vi "CalVEIN Main FRANK SFT.vi"() -> ()   [LabVIEW 2016]
uses:
  Type Defs/Sensor Data.ctl
  Type Defs/Boxcar.ctl
  Control 1.ctl
panel:
  out "MV FUEL PT":T1="-1.97 psig"
  out "MV LOX PT":string="-1.37 psig"
  out "45% 2":string="27.30 °C"
  out "45%":string="27.40 °C"
  in  "Box cooler":bool
  out "NewVal":bool
  out "Ready To Fire Flag":bool
  out "Firing State":string[](array[string])=["System Is Not Armed", "  \n", " ", " ", " ", " ", " ", " "]
  in  "Arm Flag":bool
  in  "Sample Rate (secs)":u32=1000
  out "Burn Time\nCountdown (secs)":string="0.00"
  out "Boxcar Data":T2={"AI Sensor Data"={"Sensor Array"=[{"Description"="MV FUEL PT", "Last Reading"="-1.37", "Coefs"=[0.0, 5000.0], "Eng Units"="psig"}, {"Description"="MV FUEL PT", "Last Reading"="-1.97", "Coefs"=[0.0, 5000.0], "Eng Units"="psig"}, {"Description"="P1 - Chamber Pressure", "Last Reading"="-1.37", "Coefs"=[0.0, 5000.0], "Eng Units"="psig"}, {"Description"="Not Used", "Last Reading"="0.00", "Coefs"=[0.0, 0.0], "Eng Units"="psig"}, {"Description"="High Press", "Last Reading"="141.40", "Coefs"=[157.22, 50099.0], "Eng Units"="psig"}, {"Description"="Not Use", "Last Reading"="0.00", "Coefs"=[0.0, 0.0], "Eng Units"="psig"}, {"Description"="Load Cell", "Last Reading"="-5.59", "Coefs"=[-8.51, -8297.0], "Eng Units"="lb"}, {"Description"="CHAMBER", "Last Reading"="-0.98", "Coefs"=[0.0, 5000.0], "Eng Units"="psig"}, {"Description"="P6 - GHE Fill Pressure", "Last Reading"="-0.32", "Coefs"=[0.0, 5000.0], "Eng Units"="psig"}, {"Description"="P8 - Pneumatics Pressure", "Last Reading"="-0.78", "Coefs"=[0.0, 5000.0], "Eng Units"="psig"}, {"Description"="Not Used", "Last Reading"="0.00", "Coefs"=[0.0, 0.0], "Eng Units"=""}, {"Description"="Not Used", "Last Reading"="0.00", "Coefs"=[0.0, 0.0], "Eng Units"=""}, {"Description"="Not Used", "Last Reading"="0.00", "Coefs"=[0.0, 0.0], "Eng Units"=""}, {"Description"="Not Used", "Last Reading"="0.00", "Coefs"=[0.0, 0.0], "Eng Units"=""}, {"Description"="Not Used", "Last Reading"="0.00", "Coefs"=[0.0, 0.0], "Eng Units"=""}, {"Description"="Not Used", "Last Reading"="0.00", "Coefs"=[0.0, 0.0], "Eng Units"=""}, {"Description"="QD Sep Indication", "Last Reading"="5.11", "Coefs"=[0.0, 1.0], "Eng Units"="On/Off"}, {"Description"="Lift Off Indicator", "Last Reading"="5.11", "Coefs"=[0.0, 1.0], "Eng Units"="On/Off"}, {"Description"="Main Valve Open Indicator", "Last Reading"="1.73", "Coefs"=[0.0, 1.0], "Eng Units"="On/Off"}, {"Description"="Main Valve Closed Indicator", "Last Reading"="1.68", "Coefs"=[0.0, 1.0], "Eng Units"="On/Off"}, {"Description"="Load Cell 1 - Veh Gross Weight", "Last Reading"="-17.67", "Coefs"=[-122.0, 8333.3], "Eng Units"="lbf"}, {"Description"="Load Cell 2 - - Veh Gross Weight", "Last Reading"="-2.48", "Coefs"=[0.0, 8333.33], "Eng Units"="lbf"}, {"Description"="Not Used", "Last Reading"="0.00", "Coefs"=[0.0, 0.0], "Eng Units"=""}, {"Description"="Not Used", "Last Reading"="0.00", "Coefs"=[0.0, 0.0], "Eng Units"=""}, {"Description"="LOX TANK SFT ", "Last Reading"="-126.56", "Coefs"=[-126.49, 245.99], "Eng Units"="psi"}, {"Description"="FUEL TANK SFT ", "Last Reading"="-126.56", "Coefs"=[-126.49, 245.99], "Eng Units"="psi"}, {"Description"="DOME SET SFT", "Last Reading"="-126.56", "Coefs"=[-126.49, 245.99], "Eng Units"="psi"}, {"Description"="", "Last Reading"="0.00", "Coefs"=[], "Eng Units"=""}, {"Description"="", "Last Reading"="0.00", "Coefs"=[], "Eng Units"=""}, {"Description"="", "Last Reading"="0.00", "Coefs"=[], "Eng Units"=""}, {"Description"="", "Last Reading"="0.00", "Coefs"=[], "Eng Units"=""}, {"Description"="", "Last Reading"="0.00", "Coefs"=[], "Eng Units"=""}]}, "TC Array"=[27.395629361000005, 27.395629361000005, 27.395629361000005, 27.2964472325, 27.494811489499995, 27.395629361000005, 27.395629361000005, 1369.6815, 1369.6815, 1369.6815, 1369.6815, 1369.6815, 1369.6815, 1369.6815]}
  out "?":string="-0.32 psig"
  out "Log Refnum":refnum<file>
  out "Log Epoch":u32
  out "Log Number":i32=279
  in  "Data Log Flag":bool
  out "File Path":path
  out "Eng Data & Units":string[](array[string])=["-1.37 psig", "-1.97 psig", "-1.33 psig", "0.00 psig", "141.40 psig", "0.00 psig", "-5.59 lb", "-0.98 psig", "-0.32 psig", "-0.73 psig", "0.00 ", "0.00 ", "0.00 ", "0.00 ", "0.00 ", "0.00 ", "5.10 On/Off", "5.11 On/Off", "1.73 On/Off", "1.69 On/Off", "-17.67 lbf", "-2.48 lbf", "0.00 ", "0.00 ", "-126.56 psi", "-126.56 psi", "-126.56 psi", "0.00 ", "0.00 ", "0.00 ", "0.00 ", "0.00 "]
  out "TC String Array":string[](array[string])=["27.40 °C", "27.40 °C", "27.40 °C", "27.30 °C", "27.49 °C", "27.40 °C", "27.40 °C", "1369.68 °C", "1369.68 °C", "1369.68 °C", "1369.68 °C", "1369.68 °C", "1369.68 °C", "1369.68 °C"]
  in  "Data Log Button":bool
  in  "Sequence Abort":bool
  out "Igniter Abort":bool
  out "Elapsed Time":u32=10554
  in  "Auto Sequence":bool
  in  "Auto Sequence Flag":bool
  out "Epoch":u32=5746771
  out "Countdown (secs)":i32
  in  "MV Open Start":dbl
  in  "Burn Time":dbl=300.0
  in  "Igniter Start":dbl=-3.0
  in  "Countdown":dbl=-10.0
  in  "Igniter Minimum\nTemp (°C)":dbl=100.0
  in  "Auto Switch":bool
  out "?":string="1369.68 °C"
  out "Thermometer 2":dbl(slide)=1369.6815 scale=0.0..1000.0
  out "Thermometer":dbl(slide)=1369.6815 scale=0.0..1000.0
  out "Igniter Temp (°C)":string="1369.68 °C"
  out "?":string="27.40 °C"
  out "30%":string="27.40 °C"
  out "QD Sep Indicator":bool=TRUE
  out "Liftoff Indicator":bool=TRUE
  out "MV Closed Ind":bool
  out "MV Open Ind":bool
  out "Load Cell":string="-5.59 lb"
  out "?":string="-0.73 psig"
  out "?":string="-0.98 psig"
  out "?":string="-126.56 psi"
  out "?":string="141.40 psig"
  out "?":string="-0.98 psig"
  out "P3":string="-126.56 psi"
  in  "High Press":bool
  in  "High Press Vent":bool
  in  "MV Open":bool
  in  "MV Closed":bool
  out "P2":string="-126.56 psi"
  in  "Remote QD Sep":bool
  in  "GHe Fill":bool
  in  "Igniter Pwr":bool
  in  "Dome Set":bool
  in  "Dome Vent":bool
  in  "Fuel Vent":bool
  in  "LOX Vent":bool
  out "Relay States":bool[](array[boolean])
  in  "stop":bool
  in  "AI Sensor Data":T3={"Sensor Array"=[{"Description"="MV FUEL PT", "Last Reading"="-1.37", "Coefs"=[0.0, 5000.0], "Eng Units"="psig"}, {"Description"="MV FUEL PT", "Last Reading"="-1.97", "Coefs"=[0.0, 5000.0], "Eng Units"="psig"}, {"Description"="P1 - Chamber Pressure", "Last Reading"="-1.33", "Coefs"=[0.0, 5000.0], "Eng Units"="psig"}, {"Description"="Not Used", "Last Reading"="0.00", "Coefs"=[0.0, 0.0], "Eng Units"="psig"}, {"Description"="High Press", "Last Reading"="141.40", "Coefs"=[157.22, 50099.0], "Eng Units"="psig"}, {"Description"="Not Use", "Last Reading"="0.00", "Coefs"=[0.0, 0.0], "Eng Units"="psig"}, {"Description"="Load Cell", "Last Reading"="-5.59", "Coefs"=[-8.51, -8297.0], "Eng Units"="lb"}, {"Description"="CHAMBER", "Last Reading"="-0.98", "Coefs"=[0.0, 5000.0], "Eng Units"="psig"}, {"Description"="P6 - GHE Fill Pressure", "Last Reading"="-0.32", "Coefs"=[0.0, 5000.0], "Eng Units"="psig"}, {"Description"="P8 - Pneumatics Pressure", "Last Reading"="-0.73", "Coefs"=[0.0, 5000.0], "Eng Units"="psig"}, {"Description"="Not Used", "Last Reading"="0.00", "Coefs"=[0.0, 0.0], "Eng Units"=""}, {"Description"="Not Used", "Last Reading"="0.00", "Coefs"=[0.0, 0.0], "Eng Units"=""}, {"Description"="Not Used", "Last Reading"="0.00", "Coefs"=[0.0, 0.0], "Eng Units"=""}, {"Description"="Not Used", "Last Reading"="0.00", "Coefs"=[0.0, 0.0], "Eng Units"=""}, {"Description"="Not Used", "Last Reading"="0.00", "Coefs"=[0.0, 0.0], "Eng Units"=""}, {"Description"="Not Used", "Last Reading"="0.00", "Coefs"=[0.0, 0.0], "Eng Units"=""}, {"Description"="QD Sep Indication", "Last Reading"="5.10", "Coefs"=[0.0, 1.0], "Eng Units"="On/Off"}, {"Description"="Lift Off Indicator", "Last Reading"="5.11", "Coefs"=[0.0, 1.0], "Eng Units"="On/Off"}, {"Description"="Main Valve Open Indicator", "Last Reading"="1.73", "Coefs"=[0.0, 1.0], "Eng Units"="On/Off"}, {"Description"="Main Valve Closed Indicator", "Last Reading"="1.69", "Coefs"=[0.0, 1.0], "Eng Units"="On/Off"}, {"Description"="Load Cell 1 - Veh Gross Weight", "Last Reading"="-17.67", "Coefs"=[-122.0, 8333.3], "Eng Units"="lbf"}, {"Description"="Load Cell 2 - - Veh Gross Weight", "Last Reading"="-2.48", "Coefs"=[0.0, 8333.33], "Eng Units"="lbf"}, {"Description"="Not Used", "Last Reading"="0.00", "Coefs"=[0.0, 0.0], "Eng Units"=""}, {"Description"="Not Used", "Last Reading"="0.00", "Coefs"=[0.0, 0.0], "Eng Units"=""}, {"Description"="LOX TANK SFT ", "Last Reading"="-126.56", "Coefs"=[-126.49, 245.99], "Eng Units"="psi"}, {"Description"="FUEL TANK SFT ", "Last Reading"="-126.56", "Coefs"=[-126.49, 245.99], "Eng Units"="psi"}, {"Description"="DOME SET SFT", "Last Reading"="-126.56", "Coefs"=[-126.49, 245.99], "Eng Units"="psi"}, {"Description"="", "Last Reading"="0.00", "Coefs"=[], "Eng Units"=""}, {"Description"="", "Last Reading"="0.00", "Coefs"=[], "Eng Units"=""}, {"Description"="", "Last Reading"="0.00", "Coefs"=[], "Eng Units"=""}, {"Description"="", "Last Reading"="0.00", "Coefs"=[], "Eng Units"=""}, {"Description"="", "Last Reading"="0.00", "Coefs"=[], "Eng Units"=""}]}
  # "CSULB Launch Team Control System"
  # "Questions regrads this system please direct them to Thanh Truc Le truclee126@gmail.com"
  # "Autosequence\n Parameters"
  # "30%"
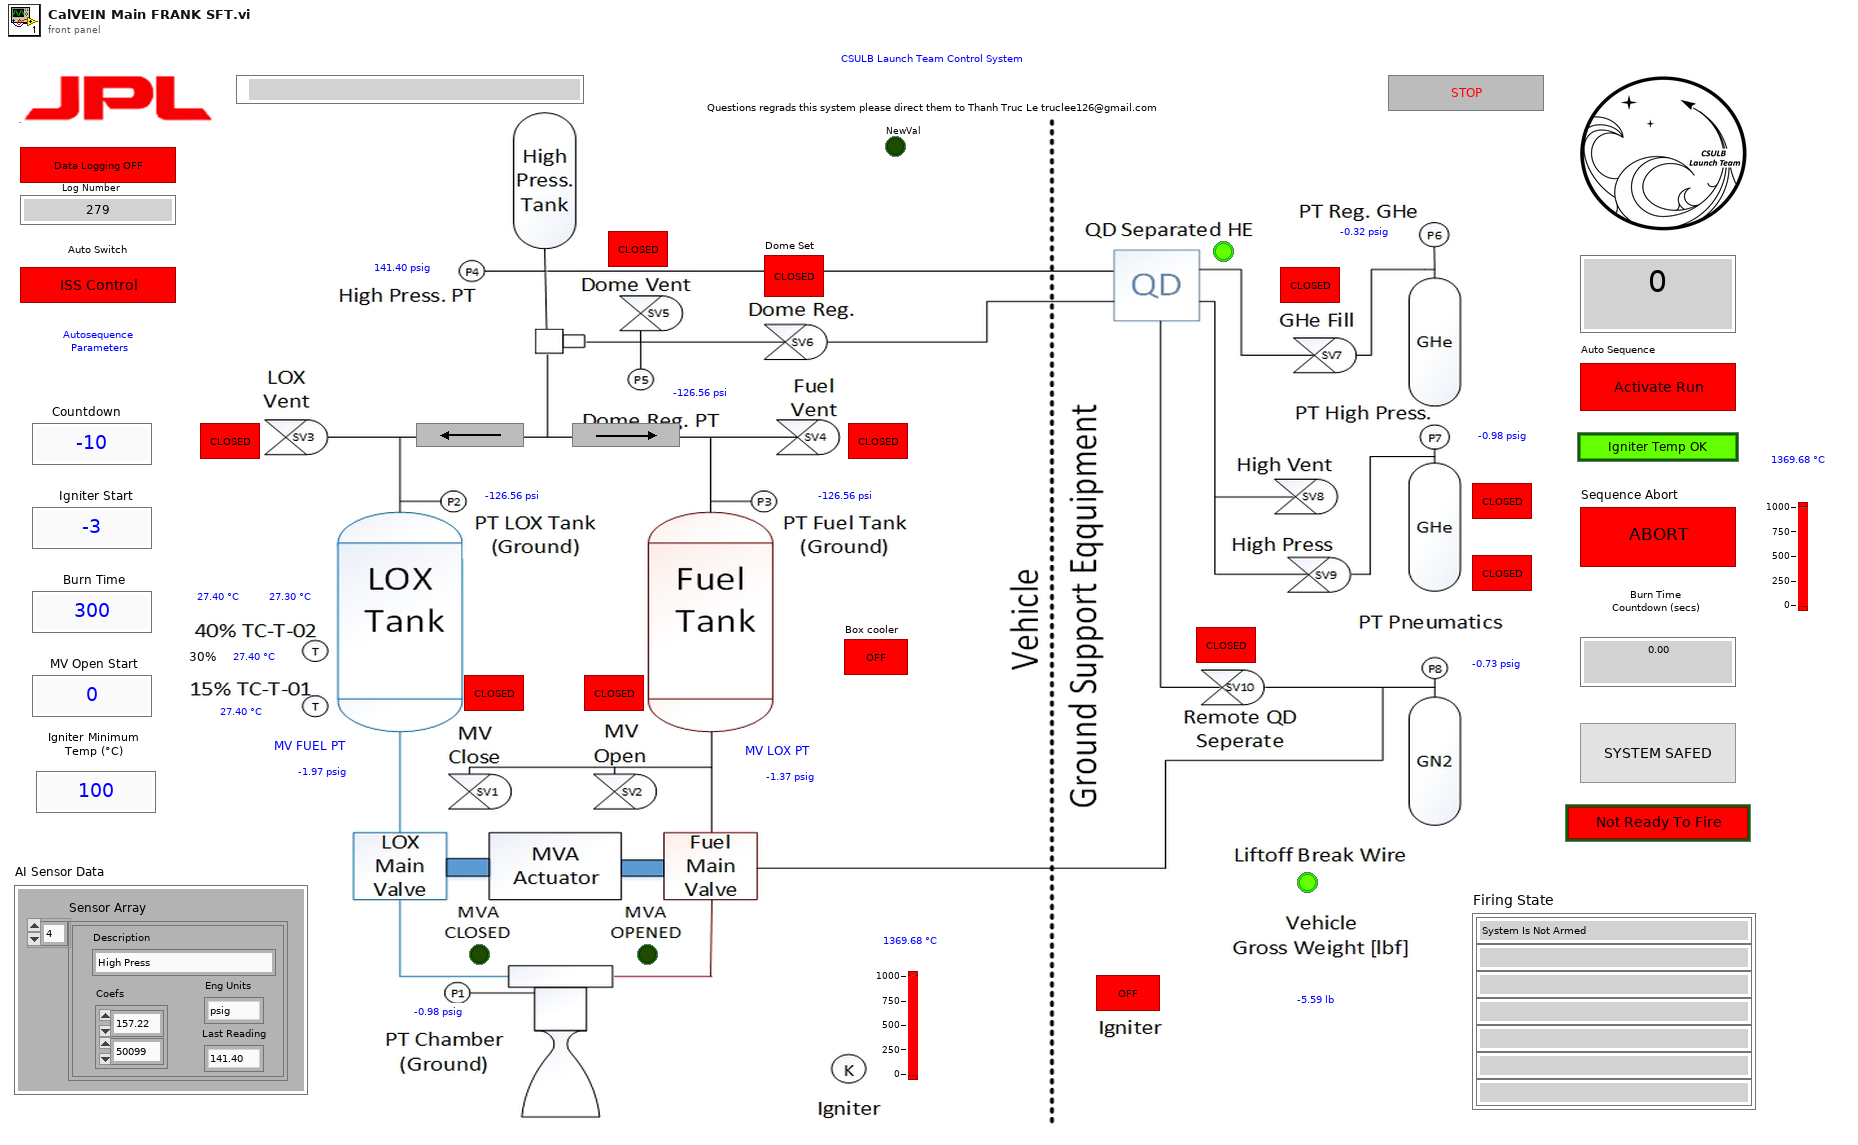
[diagram p1: front panel]
types:
  T1 = typedef "Control 1.ctl" = string
  T2 = typedef "Boxcar.ctl" = cluster{"AI Sensor Data":T3, "TC Array":dbl[]}
  T3 = typedef "Sensor Data.ctl" = cluster{"Sensor Array":cluster{"Description":string, "Last Reading":string, "Coefs":dbl[], "Eng Units":string}[]}
  T4 = cluster{"Description":string, "Last Reading":string, "Coefs":dbl[], "Eng Units":string}[]
  T5 = enum16{"open", "replace", "create", "open or create", "replace or create", "replace or create with confirmation"}
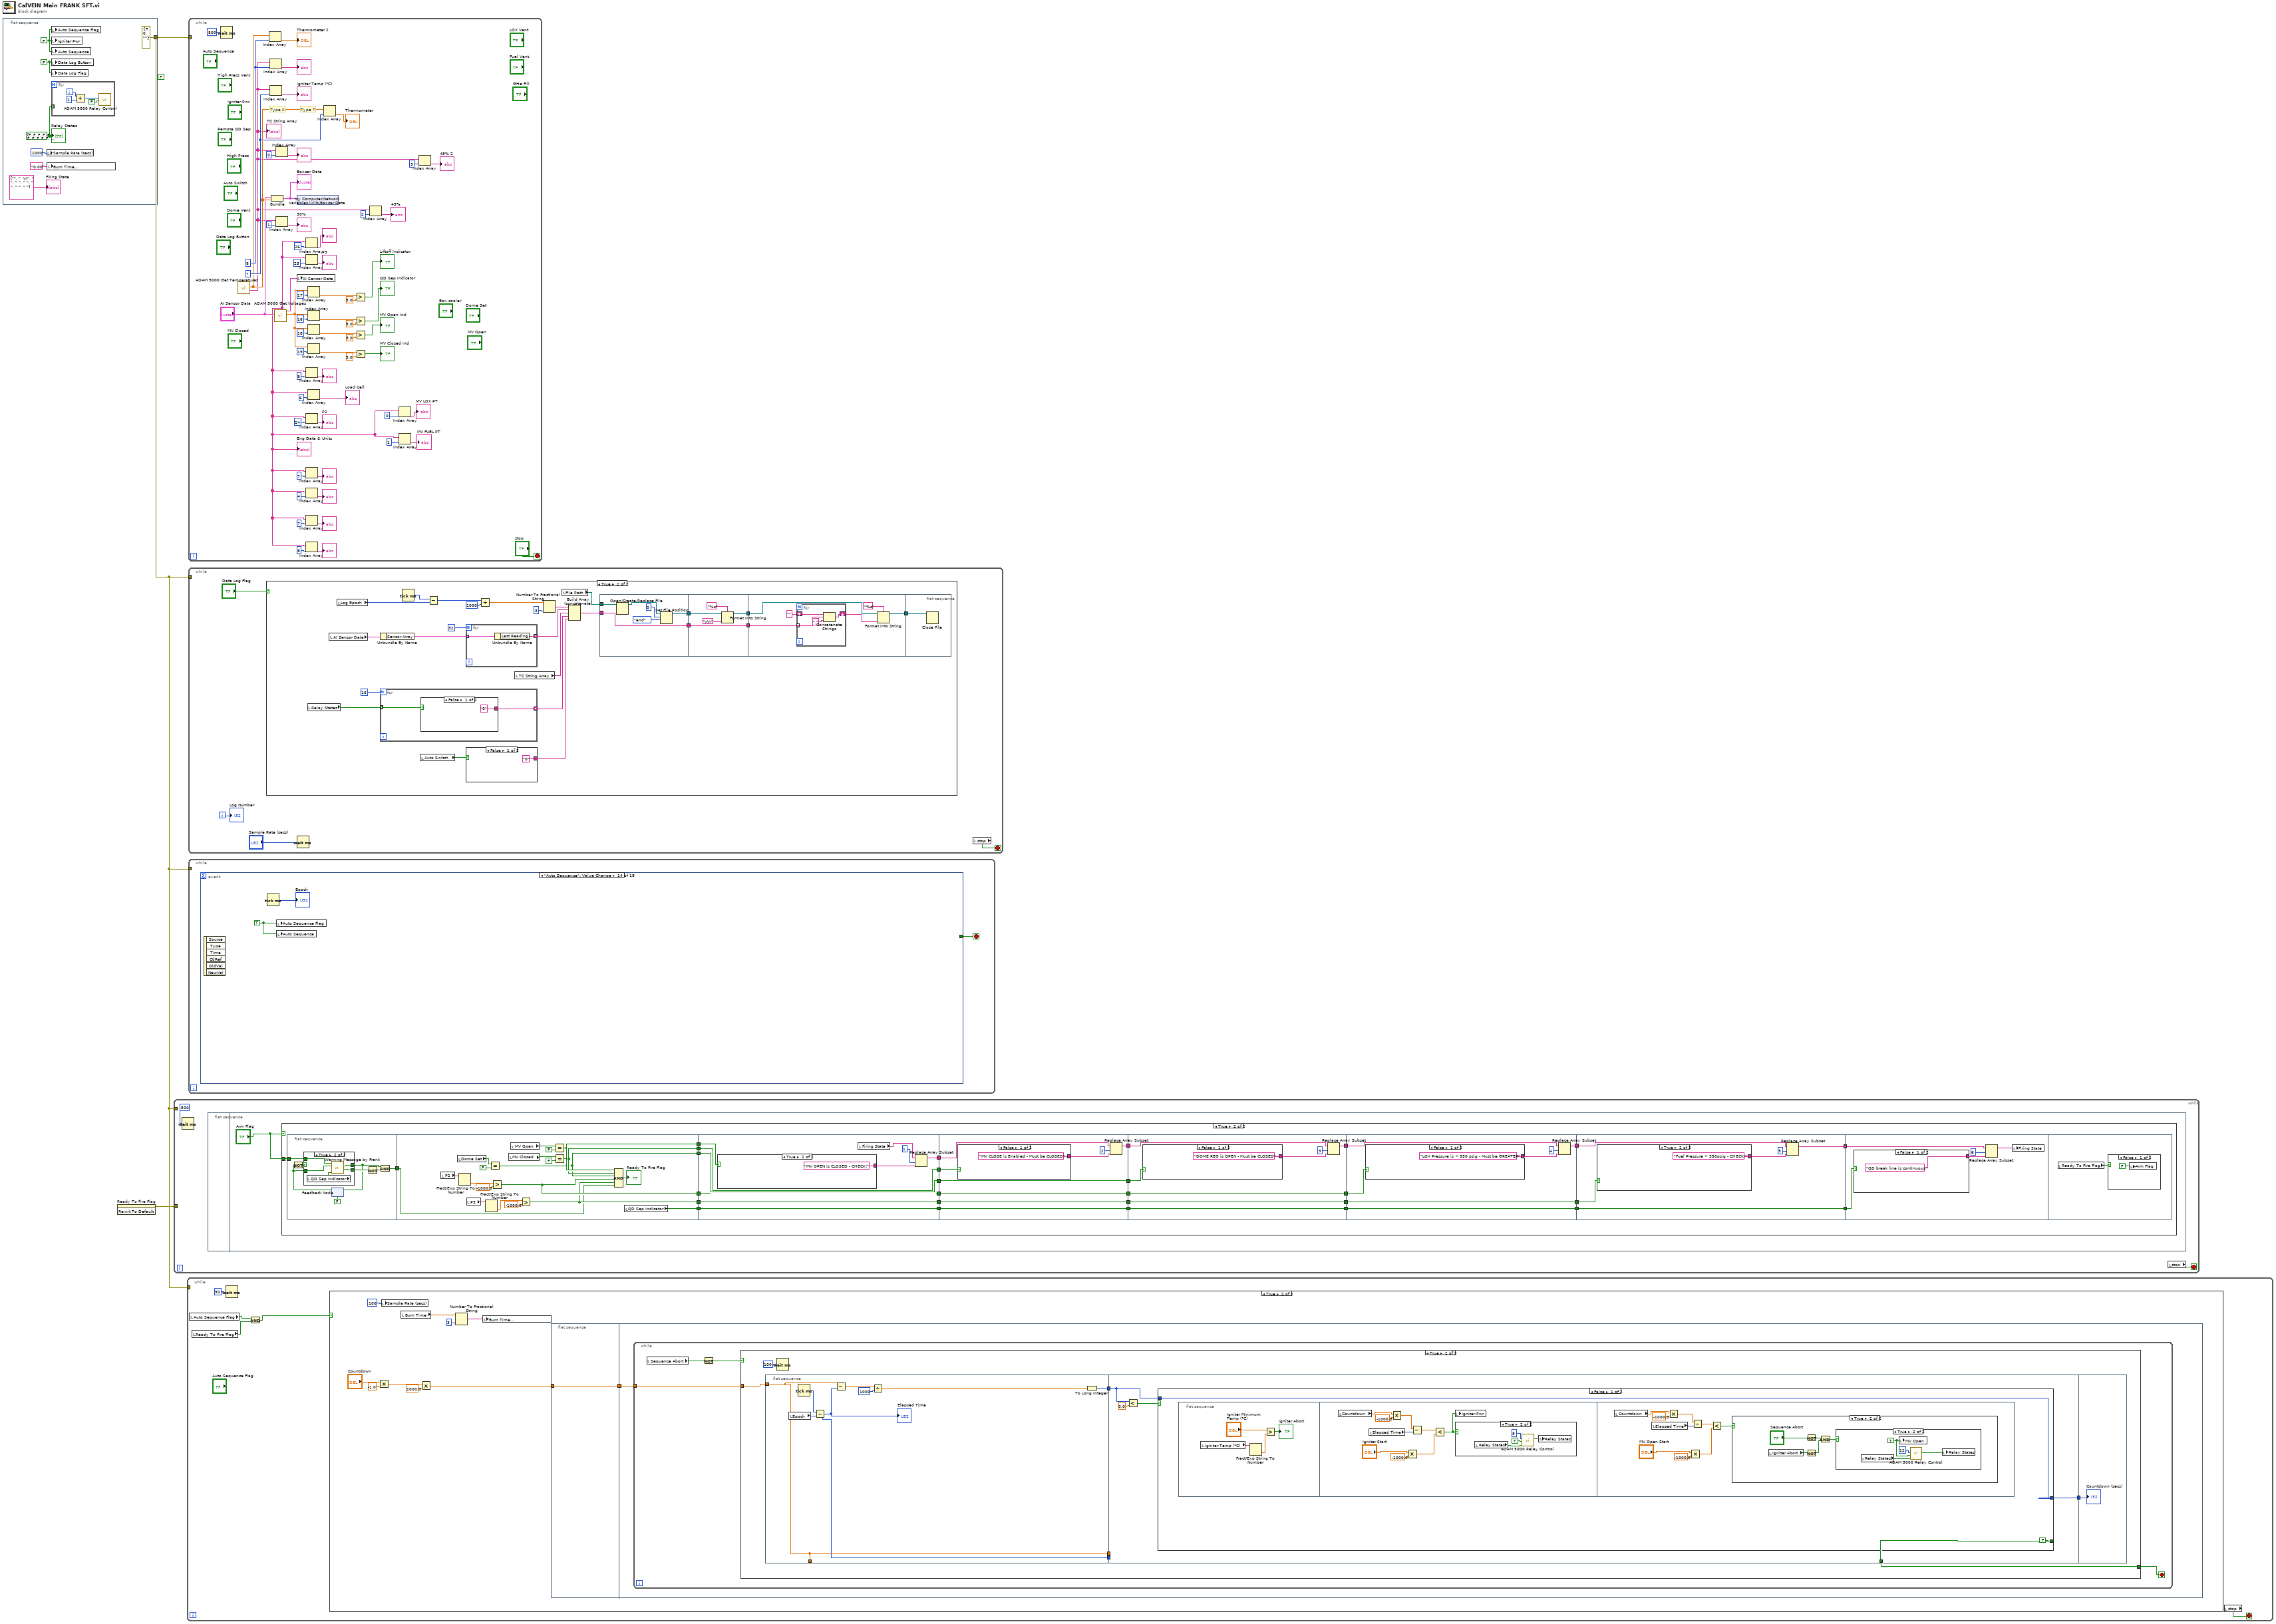
[diagram p0: block diagram]
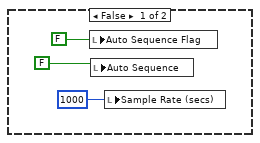
[diagram p2: hidden frame]
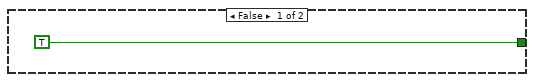
[diagram p3: hidden frame]
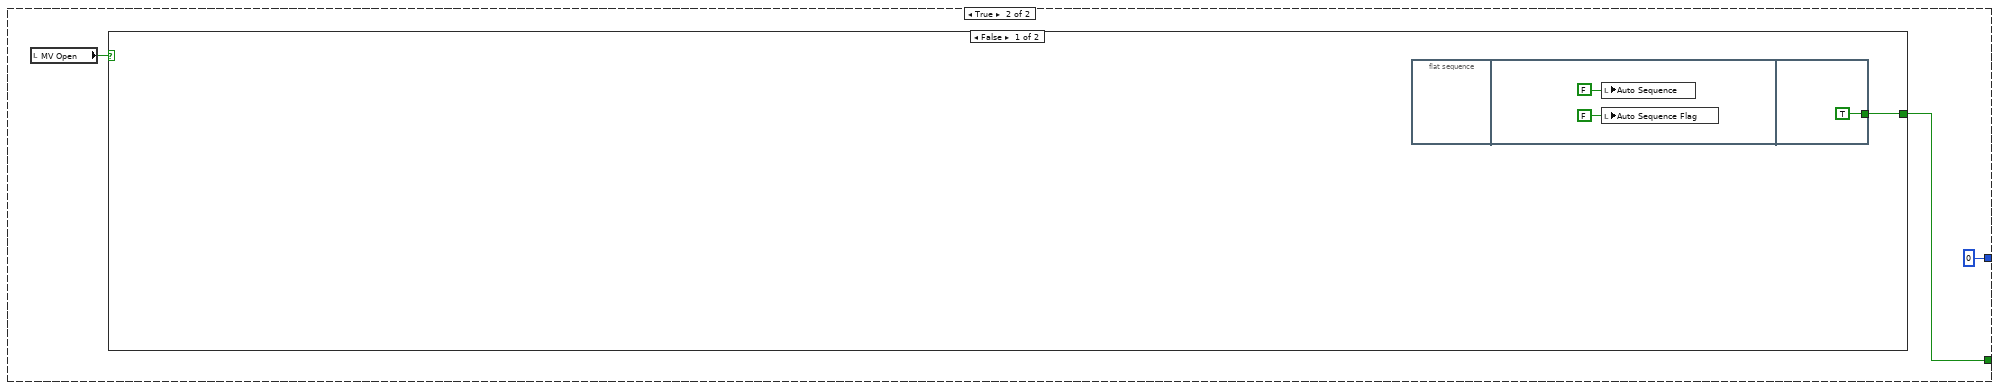
[diagram p7: hidden frame]
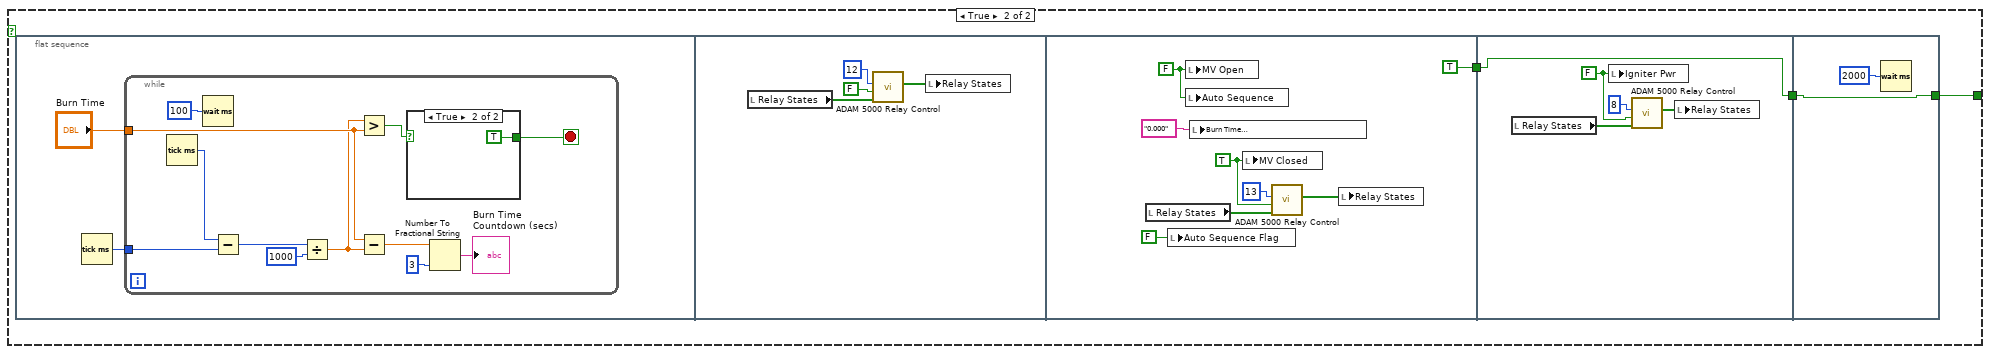
[diagram p8: hidden frame]
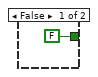
[diagram p9: hidden frame]
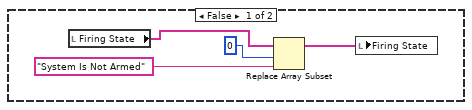
[diagram p10: hidden frame]
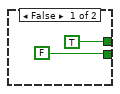
[diagram p11: hidden frame]
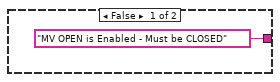
[diagram p12: hidden frame]
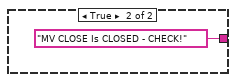
[diagram p13: hidden frame]
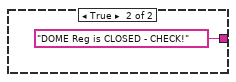
[diagram p14: hidden frame]
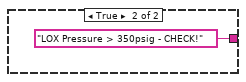
[diagram p15: hidden frame]
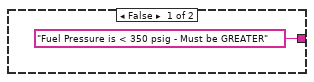
[diagram p16: hidden frame]
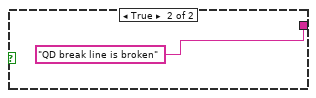
[diagram p17: hidden frame]
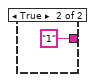
[diagram p20: hidden frame]
diagram:
  (unwired) FALSE
  n1 = flat-sequence {
    tunnel: [errorcluster {"status"=FALSE, "code"=0, "source"=""} ("error constant")] -> w2
    frame #0 {
      w6 = FALSE ("Data Lof Flag")
      w7 = FALSE ("Auto Sequence Flag")
      w8 = bool[] [FALSE, FALSE, FALSE, FALSE, FALSE, FALSE, FALSE, FALSE, FALSE, FALSE, FALSE, FALSE, FALSE, FALSE, FALSE, FALSE]
      n2 = local write "Sample Rate (secs)"(u32 1000 ("Sample Rate (secs)")) -> ()
      n3 = local write "Burn Time\nCountdown (secs)"("0.00" ("Burn Time\nCountdown (secs)")) -> ()
      n4 = local write "Auto Sequence Flag"(w7) -> ()
      n5 = local write "Igniter Pwr"(w7) -> ()
      n6 = local write "Auto Sequence"(w7) -> ()
      n7 = local write "Data Log Button"(w6) -> ()
      n8 = local write "Data Log Flag"(w6) -> ()
      n9 = for {
        tunnel: w8 -> [_] mode=indexing
        i -> [w13]
        n10 = Add(x=w13, y=1) -> (x+y=w11:i32)
        n11 = call "ADAM 5000 Relay Control.vi"("State"=FALSE, "Relay # (1=1st relay)"=w11) -> ()  [unwired: 9 in, 1 out]
      }
      "Relay States" <- w8
      "Firing State" <- string[] ["", "  \n", " ", " ", " ", " ", " ", " "]
    }
  }
  n12 = invoke on="Ready To Fire Flag" class="Bool (strict)" method="Reinit To Default"() -> (error out=w1:errorcluster)  [unwired: 3 in, 2 out]
  n13 = while {
    tunnel: w2 -> [_]
    tunnel: w1 -> [_]
    stop <- w14 stop-if-true
    n14 = Wait (ms)(milliseconds to wait=u32 500) -> ()  [unwired: 1 out]
    n15 = flat-sequence {
      frame #0 {
      }
      frame #1 {
        n16 = case shown="True" "Arm Flag" {
          tunnel: "Arm Flag" -> [_ w28]
          frame False {
            n17 = local read "Firing State"() -> (w20:string[])
            n18 = Replace Array Subset(array=w20, new element="System Is Not Armed" ("new element/subarray"), index=0) -> (w17:string[])
            n19 = local write "Firing State"(w17) -> ()
          }
          frame True {
            n20 = flat-sequence {
              tunnel: w28 -> [w56]
              tunnel: [w49] -> w27
              tunnel: [w71] -> w48
              tunnel: [w70] -> w46
              tunnel: [w69] -> w42
              tunnel: [w68] -> w36
              tunnel: [w67] -> w31
              tunnel: w27 -> [w65]
              tunnel: [w64] -> w21
              tunnel: w48 -> [w93]
              tunnel: [w89] -> w47
              tunnel: w46 -> [w89]
              tunnel: [w88] -> w45
              tunnel: [w87] -> w43
              tunnel: w42 -> [w87]
              tunnel: [w86] -> w37
              tunnel: w36 -> [w86]
              tunnel: [w85] -> w32
              tunnel: w31 -> [w85]
              tunnel: [w84] -> w22
              tunnel: w21 -> [w84]
              tunnel: w47 -> [w102]
              tunnel: w45 -> [w101]
              tunnel: [w100] -> w44
              tunnel: w43 -> [w100]
              tunnel: [w99] -> w41
              tunnel: [w98] -> w38
              tunnel: w37 -> [w98]
              tunnel: [w97] -> w33
              tunnel: w32 -> [w97]
              tunnel: [w96] -> w23
              tunnel: w22 -> [w96]
              tunnel: w44 -> [w112]
              tunnel: w41 -> [w111]
              tunnel: [w110] -> w40
              tunnel: [w109] -> w39
              tunnel: w38 -> [w109]
              tunnel: [w108] -> w34
              tunnel: w33 -> [w108]
              tunnel: [w107] -> w24
              tunnel: w23 -> [w107]
              tunnel: w40 -> [w121]
              tunnel: w39 -> [w120]
              tunnel: [w119] -> w35
              tunnel: w34 -> [w119]
              tunnel: [w118] -> w30
              tunnel: [w117] -> w25
              tunnel: w24 -> [w117]
              tunnel: w35 -> [w129]
              tunnel: w30 -> [w128]
              tunnel: [w127] -> w29
              tunnel: [w126] -> w26
              tunnel: w25 -> [w126]
              tunnel: w29 -> [w136]
              tunnel: w26 -> [w134]
              frame #0 {
                n21 = feedback #1(FALSE) -> (w50:bool)
                n22 = Not(x=w50) -> (.not. x?=w55:bool)
                n23 = case shown="True" w55 {
                  tunnel: w56 -> [_ w63]
                  tunnel: [FALSE w62] -> w53
                  tunnel: [TRUE w61] -> w52
                  tunnel: w50 -> [_ w60]
                  frame False {
                  }
                  frame True {
                    n24 = local read "QD Sep Indicator"() -> (w59:bool)
                    n25 = call "Warning Message by Frank.vi"("Contiuous"=w59, "ok?"=w60, "Arm Flag"=w63) -> ("super cancel"=w62:bool, "super ok"=w61:bool)  [unwired: 6 in, 1 out]
                  }
                }
                n26 = feedback-in #1(w52) -> ()
                n27 = Not(x=w53) -> (.not. x?=w54:bool)
                n28 = And(x=w52, y=w54) -> (x .and. y?=w49:bool)
              }
              frame #1 {
                n29 = local read "P2"() -> (w77:string)
                n30 = local read "Dome Set"() -> (w79:bool)
                n31 = Fract/Exp String To Number(string=w77) -> (number=w76:dbl)  [unwired: 3 in, 1 out]
                n32 = local read "P3"() -> (w72:string)
                n33 = Fract/Exp String To Number(string=w72) -> (number=w73:dbl)  [unwired: 3 in, 1 out]
                n34 = Equal?(x=w79, y=FALSE) -> (x = y?=w69:bool)
                n35 = Greater?(x=w76, y=-1000.0) -> (0:w68:bool)
                n36 = local read "MV Closed"() -> (w80:bool)
                n37 = local read "MV Open"() -> (w83:bool)
                n38 = Greater?(x=w73, y=-1000.0) -> (0:w67:bool)
                n39 = Equal?(x=w83, y=FALSE) -> (x = y?=w71:bool)
                n40 = Equal?(x=w80, y=FALSE) -> (x = y?=w70:bool)
                n41 = Compound Arithmetic op=AND(w71, w70, w69, w68, w67, w65) -> (→"Ready To Fire Flag":bool)
                n42 = local read "QD Sep Indicator"() -> (w64:bool)
              }
              frame #2 {
                n43 = case shown="True" w93 {
                  tunnel: ["MV OPEN is Enabled - Must be CLOSED" "MV OPEN Is CLOSED - CHECK!"] -> w90
                  frame False {
                  }
                  frame True {
                  }
                }
                n44 = local read "Firing State"() -> (w92:string[])
                n45 = Replace Array Subset(array=w92, new element=w90, index=1) -> (w88:string[])
              }
              frame #3 {
                n46 = case shown="False" w102 {
                  tunnel: ["MV CLOSE is Enabled - Must be CLOSED" "MV CLOSE Is CLOSED - CHECK!"] -> w104
                  frame False {
                  }
                  frame True {
                  }
                }
                n47 = Replace Array Subset(array=w101, new element=w104, index=2) -> (w99:string[])
              }
              frame #4 {
                n48 = case shown="False" w112 {
                  tunnel: ["DOME REG is OPEN - Must be CLOSED" "DOME Reg is CLOSED - CHECK!"] -> w113
                  frame False {
                  }
                  frame True {
                  }
                }
                n49 = Replace Array Subset(array=w111, new element=w113, index=3) -> (w110:string[])
              }
              frame #5 {
                n50 = case shown="False" w120 {
                  tunnel: ["LOX Pressure is < 350 psig - Must be GREATER" "LOX Pressure > 350psig - CHECK!"] -> w123
                  frame False {
                  }
                  frame True {
                  }
                }
                n51 = Replace Array Subset(array=w121, new element=w123, index=4) -> (w118:string[])
              }
              frame #6 {
                n52 = case shown="True" w129 {
                  tunnel: ["Fuel Pressure is < 350 psig - Must be GREATER" "Fuel Pressure > 350psig - CHECK!"] -> w130
                  frame False {
                  }
                  frame True {
                  }
                }
                n53 = Replace Array Subset(array=w128, new element=w130, index=5) -> (w127:string[])
              }
              frame #7 {
                n54 = case shown="False" w134 {
                  tunnel: ["QD break line is continuous" "QD break line is broken"] -> w138
                  frame False {
                  }
                  frame True {
                  }
                }
                n55 = Replace Array Subset(array=w136, new element=w138, index=6) -> (w135:string[])
                n56 = local write "Firing State"(w135) -> ()
              }
              frame #8 {
                n57 = local read "Ready To Fire Flag"() -> (w141:bool)
                n58 = case shown="False" w141 {
                  frame False {
                    n59 = local write "Arm Flag"(FALSE ("Arm Flag")) -> ()
                  }
                  frame True {
                  }
                }
              }
            }
          }
        }
      }
    }
    n60 = local read "stop"() -> (w14:bool)
  }
  n61 = while {
    tunnel: w2 -> [_]
    stop <- w147 stop-if-true
    n62 = local read "Auto Sequence Flag"() -> (w144:bool)
    n63 = local read "Ready To Fire Flag"() -> (w145:bool)
    n64 = Wait (ms)(milliseconds to wait=u32 50) -> ()  [unwired: 1 out]
    n65 = And(x=w144, y=w145) -> (x .and. y?=w143:bool)
    n66 = case shown="True" w143 {
      frame False {
        n67 = local write "Auto Sequence Flag"(FALSE ("Auto Sequence Flag")) -> ()
        n68 = local write "Auto Sequence"(FALSE ("Auto Sequence Flag")) -> ()
        n69 = local write "Sample Rate (secs)"(u32 1000 ("Sample Rate (secs)")) -> ()
      }
      frame True {
        n70 = Multiply(x="Countdown", y=-1.0) -> (x*y=w155:dbl)
        n71 = local write "Sample Rate (secs)"(u32 100 ("Sample Rate (secs)")) -> ()
        n72 = local read "Burn Time"() -> (w154:dbl)
        n73 = Multiply(x=w155, y=1000.0) -> (x*y=w159:dbl)
        n74 = Number To Fractional String(number=w154, precision (6)=i16 3) -> (F-format string=w152:string)  [unwired: 2 in]
        n75 = local write "Burn Time\nCountdown (secs)"(w152) -> ()
        n76 = flat-sequence {
          tunnel: w159 -> [w161]
          tunnel: [w161] -> w158
          tunnel: w158 -> [w162]
          frame #0 {
          }
          frame #1 {
            n77 = while {
              tunnel: w162 -> [w166]
              stop <- w163 stop-if-true
              n78 = local read "Sequence Abort"() -> (w165:bool)
              n79 = Not(x=w165) -> (.not. x?=w164:bool)
              n80 = case shown="True" w164 {
                tunnel: w166 -> [_ w170]
                tunnel: [TRUE w168] -> w163
                frame False {
                }
                frame True {
                  n81 = flat-sequence {
                    tunnel: [w177] -> _
                    tunnel: w170 -> [w177]
                    tunnel: [w178] -> w174
                    tunnel: [w177] -> w173
                    tunnel: [w175] -> w172
                    tunnel: w174 -> [_]
                    tunnel: w173 -> [_]
                    tunnel: w172 -> [w184]
                    tunnel: [w186] -> w168
                    tunnel: [w183] -> w171
                    tunnel: w171 -> [w270]
                    frame #0 {
                      n82 = local read "Epoch"() -> (w176:u32)
                      n83 = Tick Count (ms)() -> (millisecond timer value=w182:u32)
                      n84 = Subtract(x=w182, y=w176) -> (x-y=w178:u32)
                      "Elapsed Time" <- w178
                      n85 = Subtract(x=w177, y=w178) -> (x-y=w179:dbl)
                      n86 = Divide(x=w179, y=u32 1000) -> (x/y=w180:dbl)
                      n87 = To Long Integer(number=w180) -> (32bit integer=w175:i32)
                    }
                    frame #1 {
                      n88 = Less?(x=w184, y=0.0) -> (x < y?=w185:bool)
                      n89 = case shown="False" w185 {
                        tunnel: [FALSE w227] -> w186
                        tunnel: w184 -> [w188 _]
                        tunnel: [w188 0] -> w183
                        frame False {
                          n90 = flat-sequence {
                            frame #0 {
                              n91 = local read "Igniter Temp (°C)"() -> (w193:string)
                              n92 = Fract/Exp String To Number(string=w193) -> (number=w192:dbl)  [unwired: 3 in, 1 out]
                              n93 = Greater?(x="Igniter Minimum\nTemp (°C)", y=w192) -> (0:→"Igniter Abort":bool)
                            }
                            frame #1 {
                              n94 = local read "Countdown"() -> (w202:dbl)
                              n95 = local read "Elapsed Time"() -> (w199:u32)
                              n96 = Multiply(x=w202, y=-1000.0) -> (x*y=w200:dbl)
                              n97 = Multiply(x="Igniter Start", y=-1000.0) -> (x*y=w195:dbl)
                              n98 = Subtract(x=w200, y=w199) -> (x-y=w196:dbl)
                              n99 = Less?(x=w196, y=w195) -> (x < y?=w194:bool)
                              n100 = local write "Igniter Pwr"(w194) -> ()
                              n101 = case shown="True" w194 {
                                frame False {
                                }
                                frame True {
                                n102 = local read "Relay States"() -> (w204:bool[])
                                n103 = call "ADAM 5000 Relay Control.vi"("Relay States IN"=w204, "State"=TRUE, "Relay # (1=1st relay)"=8) -> ("Relay States OUT"=w203:bool[])  [unwired: 8 in]
                                n104 = local write "Relay States"(w203) -> ()
                                }
                              }
                            }
                            frame #2 {
                              n105 = local read "Countdown"() -> (w209:dbl)
                              n106 = local read "Elapsed Time"() -> (w212:u32)
                              n107 = Multiply(x=w209, y=-1000.0) -> (x*y=w211:dbl)
                              n108 = Multiply(x="MV Open Start", y=-1000.0) -> (x*y=w215:dbl)
                              n109 = Subtract(x=w211, y=w212) -> (x-y=w214:dbl)
                              n110 = Less?(x=w214, y=w215) -> (x < y?=w207:bool)
                              n111 = case shown="True" w207 {
                                frame False {
                                }
                                frame True {
                                n112 = local read "Igniter Abort"() -> (w219:bool)
                                n113 = Not(x="Sequence Abort") -> (.not. x?=w218:bool)
                                n114 = Not(x=w219) -> (.not. x?=w217:bool)
                                n115 = And(x=w218, y=w217) -> (x .and. y?=w216:bool)
                                n116 = case shown="True" w216 {
                                frame False {
                                }
                                frame True {
                                w221 = TRUE ("State")
                                n117 = local read "Relay States"() -> (w223:bool[])
                                n118 = local write "MV Open"(w221) -> ()
                                n119 = call "ADAM 5000 Relay Control.vi"("Relay States IN"=w223, "State"=w221, "Relay # (1=1st relay)"=12) -> ("Relay States OUT"=w222:bool[])  [unwired: 8 in]
                                n120 = local write "Relay States"(w222) -> ()
                                }
                                }
                                }
                              }
                            }
                          }
                        }
                        frame True {
                          n121 = local read "MV Open"() -> (w225:bool)
                          n122 = case shown="False" w225 {
                            tunnel: [w228 w234] -> w227
                            frame False {
                              n123 = flat-sequence {
                                tunnel: [TRUE] -> w228
                                frame #0 {
                                }
                                frame #1 {
                                n124 = local write "Auto Sequence"(FALSE ("Auto Sequence Flag")) -> ()
                                n125 = local write "Auto Sequence Flag"(FALSE ("Auto Sequence Flag")) -> ()
                                }
                                frame #2 {
                                }
                              }
                            }
                            frame True {
                              n126 = flat-sequence {
                                tunnel: [TRUE] -> w233
                                tunnel: w233 -> [w267]
                                tunnel: [w267] -> w232
                                tunnel: [w269] -> w234
                                tunnel: w232 -> [w269]
                                frame #0 {
                                n127 = Tick Count (ms)() -> (millisecond timer value=w235:u32)
                                n128 = while {
                                tunnel: "Burn Time" -> [w241]
                                tunnel: w235 -> [w246]
                                stop <- w242 stop-if-true
                                n129 = Tick Count (ms)() -> (millisecond timer value=w247:u32)
                                n130 = Wait (ms)(milliseconds to wait=u32 100) -> ()  [unwired: 1 out]
                                n131 = Subtract(x=w247, y=w246) -> (x-y=w245:u32)
                                n132 = Divide(x=w245, y=u32 1000) -> (x/y=w240:dbl)
                                n133 = Greater?(x=w240, y=w241) -> (0:w243:bool)
                                n134 = Subtract(x=w241, y=w240) -> (x-y=w239:dbl)
                                n135 = case shown="True" w243 {
                                tunnel: [FALSE TRUE] -> w242
                                frame False {
                                }
                                frame True {
                                }
                                }
                                n136 = Number To Fractional String(number=w239, precision (6)=i16 3) -> (F-format string=→"Burn Time\nCountdown (secs)":string)  [unwired: 2 in]
                                }
                                }
                                frame #1 {
                                n137 = local read "Relay States"() -> (w253:bool[])
                                n138 = call "ADAM 5000 Relay Control.vi"("Relay States IN"=w253, "State"=FALSE, "Relay # (1=1st relay)"=12) -> ("Relay States OUT"=w254:bool[])  [unwired: 8 in]
                                n139 = local write "Relay States"(w254) -> ()
                                }
                                frame #2 {
                                w257 = FALSE ("Auto Sequence Flag")
                                w256 = TRUE ("State")
                                n140 = local read "Relay States"() -> (w260:bool[])
                                n141 = local write "Auto Sequence Flag"(FALSE ("Auto Sequence Flag")) -> ()
                                n142 = local write "MV Open"(w257) -> ()
                                n143 = local write "Auto Sequence"(w257) -> ()
                                n144 = local write "Burn Time\nCountdown (secs)"("0.000" ("Burn Time\nCountdown (secs)")) -> ()
                                n145 = local write "MV Closed"(w256) -> ()
                                n146 = call "ADAM 5000 Relay Control.vi"("Relay States IN"=w260, "State"=w256, "Relay # (1=1st relay)"=13) -> ("Relay States OUT"=w261:bool[])  [unwired: 8 in]
                                n147 = local write "Relay States"(w261) -> ()
                                }
                                frame #3 {
                                w263 = FALSE ("State")
                                n148 = local read "Relay States"() -> (w265:bool[])
                                n149 = local write "Igniter Pwr"(w263) -> ()
                                n150 = call "ADAM 5000 Relay Control.vi"("Relay States IN"=w265, "State"=w263, "Relay # (1=1st relay)"=8) -> ("Relay States OUT"=w264:bool[])  [unwired: 8 in]
                                n151 = local write "Relay States"(w264) -> ()
                                }
                                frame #4 {
                                n152 = Wait (ms)(milliseconds to wait=u32 2000) -> ()  [unwired: 1 out]
                                }
                              }
                            }
                          }
                        }
                      }
                    }
                    frame #2 {
                      "Countdown (secs)" <- w270
                    }
                  }
                  n153 = Wait (ms)(milliseconds to wait=u32 100) -> ()  [unwired: 1 out]
                }
              }
            }
          }
        }
      }
    }
    n154 = local read "stop"() -> (w147:bool)
  }
  n155 = while {
    tunnel: w2 -> [_]
    stop <- "stop" stop-if-true
    w288 = 8 ("index")
    w291 = 7 ("index")
    # "Type T"
    # "Type K"
    n156 = Wait (ms)(milliseconds to wait=u32 500) -> ()  [unwired: 1 out]
    n157 = call "ADAM 5000 Get Temperatures.vi"() -> ("TC String Array"=w277:string[], "TC Array"=w283:dbl[])  [unwired: 10 in]
    "TC String Array" <- w277
    n158 = Index Array(array=w283, index=w288) -> (element=→"Thermometer 2":dbl)
    n159 = Index Array(array=w277, index=w288) -> (element=→"?":string)
    n160 = Index Array(array=w277, index=w291) -> (element=→"Igniter Temp (°C)":string)
    n161 = Bundle("AI Sensor Data"="AI Sensor Data", "TC Array"=w283) -> (w282:cluster{"AI Sensor Data":T3, "TC Array":dbl[]})  [unwired: 1 in]
    "Boxcar Data" <- w282
    n162 = call "ADAM 5000 Get Voltages.vi"("AI Sensor Data"="AI Sensor Data") -> ("Master Raw Data Vdc"=w297:dbl[], "AI Sensor Data Out"=w329:T3, "Eng Data & Units"=w271:string[])  [unwired: 5 in, 3 out]
    "Eng Data & Units" <- w271
    n163 = Index Array(array=w277, index=0) -> (element=→"?":string)
    n164 = Index Array(array=w277, index=1) -> (element=→"30%":string)
    n165 = shared-variable "My Computer\\Network Variables.lvlib\\Boxcar Data"(w282) -> ()  [unwired: 1 in, 1 out]
    n166 = local write "AI Sensor Data"(w329) -> ()
    n167 = Index Array(array=w271, index=26) -> (element=→"?":string)
    n168 = Index Array(array=w271, index=25) -> (element=→"P3":string)
    n169 = Index Array(array=w271, index=9) -> (element=→"?":string)
    n170 = Index Array(array=w271, index=24) -> (element=→"P2":string)
    n171 = Index Array(array=w271, index=7) -> (element=→"?":string)
    n172 = Index Array(array=w271, index=4) -> (element=→"?":string)
    n173 = Index Array(array=w271, index=7) -> (element=→"?":string)
    n174 = Index Array(array=w271, index=8) -> (element=→"?":string)
    n175 = Index Array(array=w297, index=17) -> (element=w304:dbl)
    n176 = Index Array(array=w297, index=16) -> (element=w299:dbl)
    n177 = Index Array(array=w297, index=18) -> (element=w312:dbl)
    n178 = Index Array(array=w297, index=19) -> (element=w308:dbl)
    n179 = Index Array(array=w271, index=6) -> (element=→"Load Cell":string)
    n180 = Index Array(array=w283, index=w291) -> (element=→"Thermometer":dbl)
    n181 = Greater?(x=w304, y=3.0) -> (0:→"Liftoff Indicator":bool)
    n182 = Greater?(x=w299, y=3.0) -> (0:→"QD Sep Indicator":bool)
    n183 = Greater?(x=w312, y=3.0) -> (0:→"MV Open Ind":bool)
    n184 = Greater?(x=w308, y=3.0) -> (0:→"MV Closed Ind":bool)
    n185 = Index Array(array=w277, index=2) -> (element=→"45%":string)
    n186 = Index Array(array=w271, index=0) -> (element=→"MV LOX PT":string)
    n187 = Index Array(array=w271, index=1) -> (element=→"MV FUEL PT":string)
    n188 = Index Array(array=w277, index=3) -> (element=→"45% 2":string)
  }
  n189 = while {
    tunnel: w2 -> [_]
    i -> [w333]
    stop <- w335 stop-if-true
    n190 = case shown="True" "Data Log Flag" {
      frame False {
      }
      frame True {
        n191 = local read "Relay States"() -> (w357:bool[])
        n192 = local read "AI Sensor Data"() -> (w359:T3)
        n193 = local read "Log Epoch"() -> (w350:u32)
        n194 = Unbundle By Name(w359) -> ("Sensor Array"=w358:T4)
        n195 = for {
          N: 16 -> [_]
          tunnel: w357 -> [w385] mode=indexing
          tunnel: [w384] -> w353 mode=indexing
          n196 = case shown="False" w385 {
            tunnel: ["0" "1"] -> w384
            frame False {
            }
            frame True {
            }
          }
        }
        n197 = Tick Count (ms)() -> (millisecond timer value=w351:u32)
        n198 = local read "Auto Switch"() -> (w356:bool)
        n199 = Subtract(x=w351, y=w350) -> (x-y=w349:u32)
        n200 = for {
          N: 32 -> [_]
          tunnel: w358 -> [w389] mode=indexing
          tunnel: [w388] -> w355 mode=indexing
          n201 = Unbundle By Name(w389) -> ("Last Reading"=w388:string)
        }
        n202 = case shown="False" w356 {
          tunnel: ["0" "1"] -> w352
          frame False {
          }
          frame True {
          }
        }
        n203 = Divide(x=w349, y=u32 1000) -> (x/y=w347:dbl)
        n204 = local read "TC String Array"() -> (w354:string[])
        n205 = Number To Fractional String(number=w347, precision (6)=i16 3) -> (F-format string=w345:string)  [unwired: 2 in]
        n206 = local read "File Path"() -> (w344:path)
        n207 = Build Array (concatenate)(w345, w355, w354, w353, w352) -> (w343:string[])
        n208 = flat-sequence {
          tunnel: w343 -> [w365]
          tunnel: w344 -> [w364]
          tunnel: [w365] -> w341
          tunnel: [w360] -> w338
          tunnel: [w366] -> w342
          tunnel: w341 -> [w370]
          tunnel: [w370] -> w340
          tunnel: w338 -> [w367]
          tunnel: w342 -> [w373]
          tunnel: w340 -> [w376]
          tunnel: [w371] -> w339
          tunnel: w339 -> [w381]
          frame #0 {
            n209 = Open/Create/Replace File(file path (use dialog)=w364) -> (refnum out=w363:refnum<file>)  [unwired: 5 in, 2 out]
            n210 = Set File Position(offset (in bytes) (0)=i64 0, refnum=w363, from (0:start)=enum16{"start", "end", "current"}."end") -> (refnum out=w360:refnum<file>)  [unwired: 1 in, 1 out]
          }
          frame #1 {
            n211 = Format Into String(format string="%s", initial string=w367, "\r\n") -> (resulting string=w366:refnum<file>)  [unwired: 1 in, 1 out]
          }
          frame #2 {
            n212 = for {
              shift-right: [w378] -> w372
              shift-left: "" -> [w377]
              tunnel: w376 -> [w380] mode=indexing
              n213 = Concatenate Strings(w377, w380, "," ("string")) -> (w378:string)
            }
            n214 = Format Into String(format string="%s", initial string=w373, w372) -> (resulting string=w371:refnum<file>)  [unwired: 1 in, 1 out]
          }
          frame #3 {
            n215 = Close File(refnum=w381) -> ()  [unwired: 1 in, 2 out]
          }
        }
      }
    }
    n216 = Wait (ms)(milliseconds to wait="Sample Rate (secs)") -> ()  [unwired: 1 out]
    n217 = local read "stop"() -> (w335:bool)
    "Log Number" <- w333
  }
  n218 = while {
    tunnel: w2 -> [_]
    stop <- w390 stop-if-true
    n219 = event shown="[13] \"Auto Sequence\": Value Change" {
      selector: _ -> [_ _ _ _ _ _ _ _ _ _ _ _ _ _ _ _ _ _]
      dyn-events: _ -> [_ _ _ _ _ _ _ _ _ _ _ _ _ _ _ _ _ _]
      timeout: _ -> [_ _ _ _ _ _ _ _ _ _ _ _ _ _ _ _ _ _]
      tunnel: [_ _ _ _ _ _ _ _ w419 _ _ _ _ _ _ _ _ _] -> w390
      event Timeout {
        n220 = event-data() -> ()  [unwired: 1 in, 3 out]
      }
      event "LOX Vent": Value Change {
        n221 = event-data() -> ("NewVal"=w393:bool)  [unwired: 1 in, 5 out]
        n222 = local read "Relay States"() -> (w392:bool[])
        n223 = call "ADAM 5000 Relay Control.vi"("Relay States IN"=w392, "State"=w393, "Relay # (1=1st relay)"=1) -> ("Relay States OUT"=w391:bool[])  [unwired: 8 in]
        n224 = local write "Relay States"(w391) -> ()
      }
      event "Fuel Vent": Value Change {
        n225 = event-data() -> ("NewVal"=w395:bool)  [unwired: 1 in, 5 out]
        n226 = local read "Relay States"() -> (w397:bool[])
        n227 = call "ADAM 5000 Relay Control.vi"("Relay States IN"=w397, "State"=w395, "Relay # (1=1st relay)"=2) -> ("Relay States OUT"=w396:bool[])  [unwired: 8 in]
        n228 = local write "Relay States"(w396) -> ()
      }
      event "Dome Vent": Value Change {
        n229 = event-data() -> ("NewVal"=w399:bool)  [unwired: 1 in, 5 out]
        n230 = local read "Relay States"() -> (w401:bool[])
        n231 = call "ADAM 5000 Relay Control.vi"("Relay States IN"=w401, "State"=w399, "Relay # (1=1st relay)"=6) -> ("Relay States OUT"=w400:bool[])  [unwired: 8 in]
        n232 = local write "Relay States"(w400) -> ()
      }
      event "Dome Set": Value Change {
        n233 = event-data() -> ("NewVal"=w403:bool)  [unwired: 1 in, 5 out]
        n234 = local read "Relay States"() -> (w405:bool[])
        n235 = call "ADAM 5000 Relay Control.vi"("Relay States IN"=w405, "State"=w403, "Relay # (1=1st relay)"=5) -> ("Relay States OUT"=w404:bool[])  [unwired: 8 in]
        n236 = local write "Relay States"(w404) -> ()
      }
      event "Igniter Pwr": Value Change {
        n237 = event-data() -> ("NewVal"=w407:bool)  [unwired: 1 in, 5 out]
        n238 = local read "Relay States"() -> (w409:bool[])
        n239 = call "ADAM 5000 Relay Control.vi"("Relay States IN"=w409, "State"=w407, "Relay # (1=1st relay)"=8) -> ("Relay States OUT"=w408:bool[])  [unwired: 8 in]
        n240 = local write "Relay States"(w408) -> ()
      }
      event "GHe Fill": Value Change {
        n241 = event-data() -> ("NewVal"=w411:bool)  [unwired: 1 in, 5 out]
        n242 = local read "Relay States"() -> (w413:bool[])
        n243 = call "ADAM 5000 Relay Control.vi"("Relay States IN"=w413, "State"=w411, "Relay # (1=1st relay)"=9) -> ("Relay States OUT"=w412:bool[])  [unwired: 8 in]
        n244 = local write "Relay States"(w412) -> ()
      }
      event "Remote QD Sep": Value Change {
        n245 = event-data() -> ("NewVal"=w415:bool)  [unwired: 1 in, 5 out]
        n246 = local read "Relay States"() -> (w417:bool[])
        n247 = call "ADAM 5000 Relay Control.vi"("Relay States IN"=w417, "State"=w415, "Relay # (1=1st relay)"=10) -> ("Relay States OUT"=w416:bool[])  [unwired: 8 in]
        n248 = local write "Relay States"(w416) -> ()
      }
      event "stop": Value Change {
        n249 = event-data() -> ()  [unwired: 1 in, 6 out]
        n250 = flat-sequence {
          tunnel: [TRUE] -> w419
          frame #0 {
            n251 = Wait (ms)(milliseconds to wait=u32 2000) -> ()  [unwired: 1 out]
          }
          frame #1 {
          }
        }
      }
      event "MV Closed": Value Change {
        n252 = event-data() -> ("NewVal"=w422:bool)  [unwired: 1 in, 5 out]
        n253 = local read "Relay States"() -> (w424:bool[])
        n254 = call "ADAM 5000 Relay Control.vi"("Relay States IN"=w424, "State"=w422, "Relay # (1=1st relay)"=13) -> ("Relay States OUT"=w423:bool[])  [unwired: 8 in]
        n255 = local write "Relay States"(w423) -> ()
      }
      event "High Press Vent": Value Change {
        n256 = event-data() -> ("NewVal"=w426:bool)  [unwired: 1 in, 5 out]
        n257 = local read "Relay States"() -> (w428:bool[])
        n258 = call "ADAM 5000 Relay Control.vi"("Relay States IN"=w428, "State"=w426, "Relay # (1=1st relay)"=15) -> ("Relay States OUT"=w427:bool[])  [unwired: 8 in]
        n259 = local write "Relay States"(w427) -> ()
      }
      event "High Press": Value Change {
        n260 = event-data() -> ("NewVal"=w430:bool)  [unwired: 1 in, 5 out]
        n261 = local read "Relay States"() -> (w432:bool[])
        n262 = call "ADAM 5000 Relay Control.vi"("Relay States IN"=w432, "State"=w430, "Relay # (1=1st relay)"=7) -> ("Relay States OUT"=w431:bool[])  [unwired: 8 in]
        n263 = local write "Relay States"(w431) -> ()
      }
      event "Auto Switch": Value Change {
        n264 = event-data() -> ("NewVal"=w435:bool)  [unwired: 1 in, 5 out]
        n265 = call "Control ETH008 Relay.vi"("On/Off"=w435, "Relay Number"=1) -> ()  [unwired: 10 in]
      }
      event "Auto Sequence": Value Change {
        w437 = TRUE ("Auto Sequence Flag")
        n266 = event-data() -> ()  [unwired: 1 in, 6 out]
        n267 = Tick Count (ms)() -> (millisecond timer value=→"Epoch":u32)
        n268 = local write "Auto Sequence Flag"(w437) -> ()
        n269 = local write "Auto Sequence"(w437) -> ()
      }
      event "Sequence Abort": Value Change {
        n270 = event-data() -> ()  [unwired: 1 in, 6 out]
        n271 = flat-sequence {
          frame #0 {
            w438 = FALSE ("Auto Sequence Flag")
            n272 = local write "Auto Sequence Flag"(w438) -> ()
            n273 = local write "Igniter Pwr"(w438) -> ()
            n274 = local write "Auto Sequence"(w438) -> ()
          }
          frame #1 {
            n275 = for {
              tunnel: bool[] [FALSE, FALSE, FALSE, FALSE, FALSE, FALSE, FALSE, FALSE, FALSE, FALSE, FALSE, FALSE, FALSE, FALSE, FALSE, FALSE] -> [_] mode=indexing
              i -> [w443]
              n276 = Add(x=w443, y=1) -> (x+y=w441:i32)
              n277 = call "ADAM 5000 Relay Control.vi"("State"=FALSE, "Relay # (1=1st relay)"=w441) -> ()  [unwired: 9 in, 1 out]
            }
          }
        }
      }
      event "Data Log Button": Value Change {
        n278 = event-data() -> ("NewVal"=w444:bool)  [unwired: 1 in, 5 out]
        n279 = case shown="True" w444 {
          frame False {
            n280 = local write "Data Log Flag"(FALSE ("Data Lof Flag")) -> ()
            n281 = local write "Data Log Flag"(FALSE ("Data Lof Flag")) -> ()
            n282 = local write "Data Log Flag"(FALSE ("Data Lof Flag")) -> ()
            n283 = local write "Data Log Flag"(FALSE ("Data Lof Flag")) -> ()
            n284 = local write "Data Log Flag"(FALSE ("Data Lof Flag")) -> ()
            n285 = local write "Data Log Flag"(FALSE ("Data Lof Flag")) -> ()
            n286 = local write "Data Log Flag"(FALSE ("Data Lof Flag")) -> ()
            n287 = local write "Data Log Flag"(FALSE ("Data Lof Flag")) -> ()
            n288 = local write "Data Log Flag"(FALSE ("Data Lof Flag")) -> ()
            n289 = local write "Data Log Flag"(FALSE ("Data Lof Flag")) -> ()
            n290 = local write "Data Log Flag"(FALSE ("Data Lof Flag")) -> ()
          }
          frame True {
            n291 = flat-sequence {
              frame #0 {
                n292 = Tick Count (ms)() -> (millisecond timer value=→"Log Epoch":u32)
                n293 = for {
                  N: 14 -> [_]
                  tunnel: [w488] -> w467 mode=indexing
                  i -> [w487]
                  n294 = Add(x=w487, y=1) -> (x+y=w485:i32)
                  n295 = Number To Fractional String(number=w485, precision (6)=i16 0) -> (F-format string=w489:string)  [unwired: 2 in]
                  n296 = Concatenate Strings("TC", w489) -> (w488:string)
                }
                n297 = for {
                  N: 16 -> [_]
                  tunnel: [w481] -> w466 mode=indexing
                  i -> [w480]
                  n298 = Add(x=w480, y=1) -> (x+y=w478:i32)
                  n299 = Number To Fractional String(number=w478, precision (6)=i16 0) -> (F-format string=w482:string)  [unwired: 2 in]
                  n300 = Concatenate Strings("Relay", w482) -> (w481:string)
                }
                n301 = local read "AI Sensor Data"() -> (w473:T3)
                n302 = Unbundle By Name(w473) -> ("Sensor Array"=w472:T4)
                n303 = for {
                  tunnel: w472 -> [w493] mode=indexing
                  tunnel: [w492] -> w470 mode=indexing
                  n304 = Unbundle By Name(w493) -> ("Description"=w492:string)
                }
                n305 = Build Array (concatenate)("Time (s)", w470, w467, w466, "Manual/Auto (1=Auto)") -> (w462:string[])
                n306 = for {
                  shift-right: [w475] -> w460
                  shift-left: "" -> [w474]
                  tunnel: w462 -> [w477] mode=indexing
                  n307 = Concatenate Strings(w474, w477, "," ("string")) -> (w475:string)
                }
                n308 = Open/Create/Replace File(operation (0:open)=T5."replace or create") -> (refnum out=w459:refnum<file>)  [unwired: 5 in, 2 out]
                "Log Refnum" <- w459
                n309 = Refnum to Path(1:w459) -> (0:→"File Path":path)
                n310 = Format Into String(format string="%s", initial string=w459, w460) -> (resulting string=w456:refnum<file>)  [unwired: 1 in, 1 out]
                n311 = Close File(refnum=w456) -> ()  [unwired: 1 in, 2 out]
              }
              frame #1 {
                n312 = Wait (ms)(milliseconds to wait=u32 1000) -> ()  [unwired: 1 out]
              }
              frame #2 {
                n313 = local write "Data Log Flag"(TRUE ("Data Lof Flag")) -> ()
              }
            }
          }
        }
      }
      event "MV Open": Value Change {
        n314 = event-data() -> ("NewVal"=w499:bool)  [unwired: 1 in, 5 out]
        "NewVal" <- w499
        n315 = local read "Relay States"() -> (w497:bool[])
        n316 = call "ADAM 5000 Relay Control.vi"("Relay States IN"=w497, "State"=w499, "Relay # (1=1st relay)"=12) -> ("Relay States OUT"=w498:bool[])  [unwired: 8 in]
        n317 = local write "Relay States"(w498) -> ()
      }
      event "Box cooler": Value Change {
        n318 = event-data() -> ("NewVal"=w500:bool)  [unwired: 1 in, 5 out]
        n319 = local read "Relay States"() -> (w502:bool[])
        n320 = call "ADAM 5000 Relay Control.vi"("Relay States IN"=w502, "State"=w500, "Relay # (1=1st relay)"=3) -> ("Relay States OUT"=w503:bool[])  [unwired: 8 in]
        n321 = local write "Relay States"(w503) -> ()
      }
    }
  }
